vi "SetConnectInfo.vi"(0 "reference in":refnum<class "DatabaseInterface.lvclass">, 5 "Connection Info":T1, 11 "error in (no error)":errorcluster) -> (4 "reference out":refnum<class "DatabaseInterface.lvclass">, 15 "error out":errorcluster)   [LabVIEW 2019, in "DatabaseInterface.lvclass"]
uses:
  DatabaseInterface.lvclass
  Database_Postgress_class/Connection Info.ctl
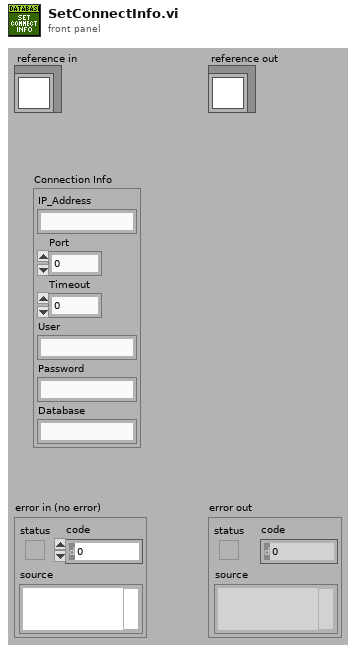
[diagram p1: front panel]
types:
  T1 = typedef "DatabaseInterface.lvclass/Connection Info.ctl" = cluster{"IP_Address":string, "Port":u16, "Timeout":i32, "User":string, "Password":string, "Database":string}
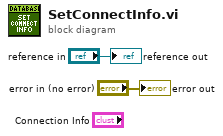
[diagram p0: block diagram]
diagram:
  "error out" <- "error in (no error)"
  "reference out" <- "reference in"
